vi "getTextFromDocument.vi"(8 "error in (no error)":errorcluster, 11 "xwpfRun in":refnum<class "xwpfRun.lvclass">) -> (0 "error out":errorcluster, 3 "xwpfRun out":refnum<class "xwpfRun.lvclass">)   [LabVIEW 2017, in "Word_Specific.lvlib" / "xwpfRun.lvclass"]
uses:
  xwpfRun.lvclass
  xwpfRun.lvclass/xwpfRun.ctl
  C:/Users/Neo/Desktop/Dev_Tools_BR/LabVIEW_NPOI/src/lib/NPOI 2.1.1/NPOI.OOXML.dll
  lib/NPOI 2.1.1/NPOI.OOXML.dll
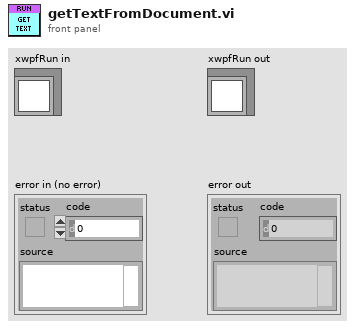
[diagram p1: front panel]
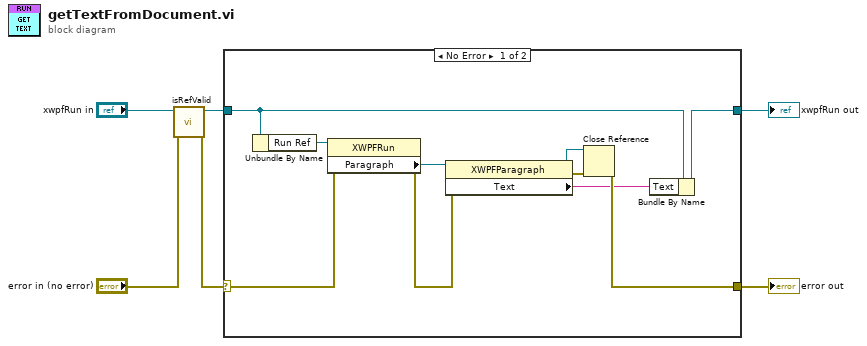
[diagram p0: block diagram]
diagram:
  n1 = call-dynamic "isRefValid.vi"("error in (no error)"="error in (no error)", "xwpfRun in"="xwpfRun in") -> ("error out"=w1:errorcluster, "xwpfRun out"=w3:refnum<class "xwpfRun.lvclass">)  [unwired: 8 in]
  n2 = case shown="No Error" w1 {
    selector: w1 -> [w16 w18]
    tunnel: [w14 w18] -> w6
    tunnel: [w15 w17] -> w4
    tunnel: w3 -> [w13 w17]
    frame No Error {
      n3 = Unbundle By Name(w13) -> ("Run Ref"=w12:refnum<k24>)
      n4 = property class="XWPFRun"(reference=w12, error in=w16) -> (error out=w10:errorcluster, "Paragraph"=w11:refnum<k24>)  [unwired: 1 out]
      n5 = property class="XWPFParagraph"(reference=w11, error in=w10) -> (reference out=w8:refnum<k24>, error out=w7:errorcluster, "Text"=w9:string)
      n6 = Close Reference(reference=w8, error in (no error)=w7) -> (error out=w14:errorcluster)
      n7 = Bundle By Name(cluster=w13, "Text"=w9) -> (w15:refnum<class "xwpfRun.lvclass">)
    }
    frame Error {
    }
  }
  "error out" <- w6
  "xwpfRun out" <- w4
